vi "ReversedEngineering UpdateClassMethods.vi"(1 "ClassPath/LvClassRef":variant, 2 "Methods":string[](array[string]), 5 "error in (no error)":errorcluster, 6 "BaseClass":bool, 7 "Don'tShowDialog(False)":bool, 8 "UseVirtualMethods(True)":bool=TRUE) -> (19 "error out":errorcluster)   [LabVIEW 2012]
uses:
  <resource>/Framework/Providers/Open_GDS/ClassProviders/Provider_BaseClassInterface/ClassReader_class/ClassReader.lvclass
  <resource>/Framework/Providers/Open_GDS/ClassProviders/Provider_LvNativeClass/ClassWriterNative_class/ClassWriterNative.lvclass
  <resource>/Framework/Providers/Open_GDS/ClassProviders/Provider_BaseClassInterface/CreateMethodData.ctl
  <resource>/Framework/Providers/Open_GDS/ClassProviders/Provider_EndevoGOOP300/GOOP300_SubVIs/GOOP300_MethodScopeType.ctl
  <resource>/Framework/Providers/Open_GDS/ClassProviders/Provider_LvNativeClass/ClassWriterNative_class/IconDetails.ctl
  <resource>/Framework/Providers/Open_GDS/ClassProviders/Provider_LvNativeClass/ClassWriterNative_class/IconSize.ctl
  <resource>/Framework/Providers/Open_GDS/ClassProviders/Provider_BaseClassInterface/ClassWriter_class/ClassWriter.lvclass
panel:
  out "Creating methods":u8(slide) scale=0.0..100.0
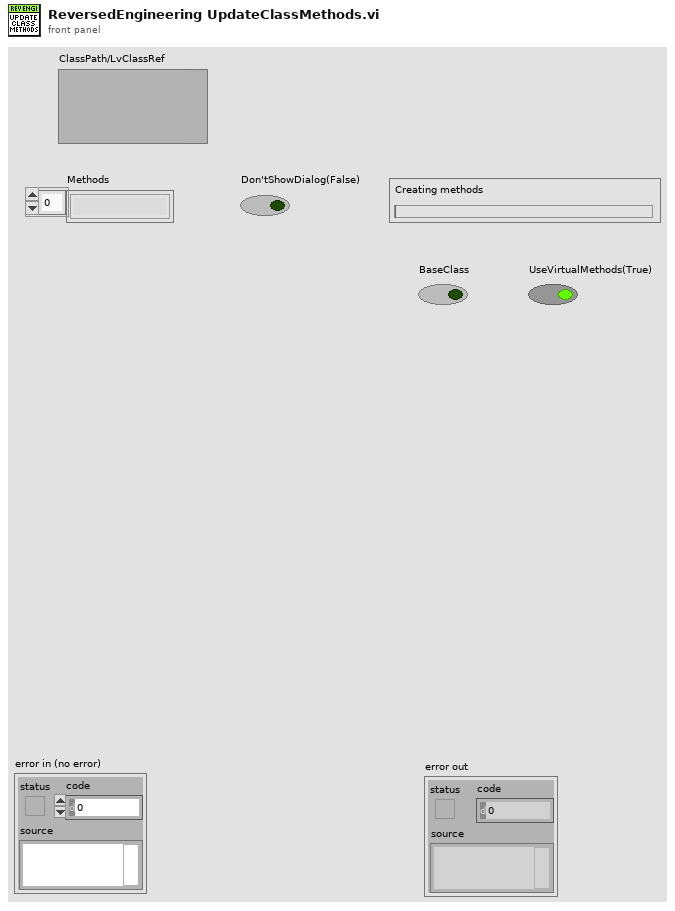
[diagram p1: front panel]
types:
  T1 = cluster{"Methods":cluster{"MethodName":string, "Private":bool, "Virtual":bool, "Reentrant":bool, "Description":string, "Icon Method Name":string, "Protected":bool, "Method Type":enum16{"Get", "Set", "GetProperty", "SetProperty"}, "Attribute":string, "ClassAtt":bool}[], "MethodPaths":path[], "MethodPrivate":bool[], "ClassItemRef":refnum<vi>}
  T2 = cluster{"MethodName":string, "Private":bool, "Virtual":bool, "Reentrant":bool, "Description":string, "Icon Method Name":string, "Protected":bool, "Method Type":enum16{"Get", "Set", "GetProperty", "SetProperty"}, "Attribute":string, "ClassAtt":bool}
  T3 = cluster{"MethodName":string, "Private":bool, "Virtual":bool, "Reentrant":bool, "Description":string, "Icon Method Name":string, "Protected":bool, "Method Type":enum16{"Get", "Set", "GetProperty", "SetProperty"}, "Attribute":string, "ClassAtt":bool}[]
  T4 = enum16{"Get", "Set", "GetProperty", "SetProperty"}
  T5 = typedef "ClassWriter.lvclass/CreateMethodData.ctl" = cluster{"MethodName":string, "RelativeMethodPath":path, "MethodDescription":string, "Scope/Visibility":T6, "MethodTemplateName":string, "IconOut":u8[][], "RelativeProjectClassPath":string, "OpenViAfterCreation":bool, "DynamicDispatchVi":bool, "ExtraCreateParameters":variant, "MustOverride":bool, "MustCallParent":bool, "IconDetails":T7, "AF-Option":variant, "TemplatePath":path}
  T6 = typedef "GOOP300_MethodScopeType.ctl" = enum16{"Use Parent Folder Scope", "Public", "Protected", "Private", "Community"}
  T7 = typedef "ClassWriterNative.lvclass/IconDetails.ctl" = cluster{"IconSize":T8, "ImageRows(32)":i32, "ConnectorPaneHeight":i32[]}
  T8 = typedef "ClassWriterNative.lvclass/IconSize.ctl" = enum16{"Full", "1 c-term high", "2 c-term high", "3 c-term high"}
  T9 = cluster{"AttributeNames":string[], "PropertyNode":bool, "FolderNames":string[]}
  T10 = typedef "ClassTypes_MethodType.ctl" = cluster{"MethodName":string, "Visibility":enum16{"Public", "Private", "Protected"}, "StereoType":string, "Path":path}
  T11 = typedef "ReversedEngineering AttributeInfoType.ctl" = cluster{"name":string, "type":T12, "dimension":i32, "typeName":string, "typePath":path, "visibility":T13}
  T12 = typedef "CommonVIs_AttributeDataType.ctl" = enum16{"UINT8", "INT8", "UINT16", "INT16", "UINT32", "INT32", "UINT64", "INT64", "SGL", "DBL", "EXT", "CSG", "CDB", "CXT", "TimeStamp", "STRING", "PATH", "BOOL", "ENUM", "RefNum", "VIRefNum", "LabVIEW Class", "Cluster", "Variant", "TypeDef", "Waveform", "LabVIEW Object", "Other", "void"}
  T13 = typedef "UMLEditor_VisibilityType.ctl" = enum16{"Public", "Private", "Protected"}
  T14 = typedef "GDSLvCLass_ClassSettingsType.ctl" = cluster{"ClassProviderName":string, "ClassTemplateUsed":string, "ClassTemplateVersion":string, "ClassDescription":string, "PlugIns":T15[], "ConnectorPanePattern":string}
  T15 = typedef "GDSLvClass_PlugIn.ctl" = cluster{"Type":T16, "ID":string, "Version":string, "Path":path, "Name":string, "Data":variant}
  T16 = typedef "GDSLvClass_PlugInTypes.ctl" = enum16{"DesignPattern", "MethodTypes"}
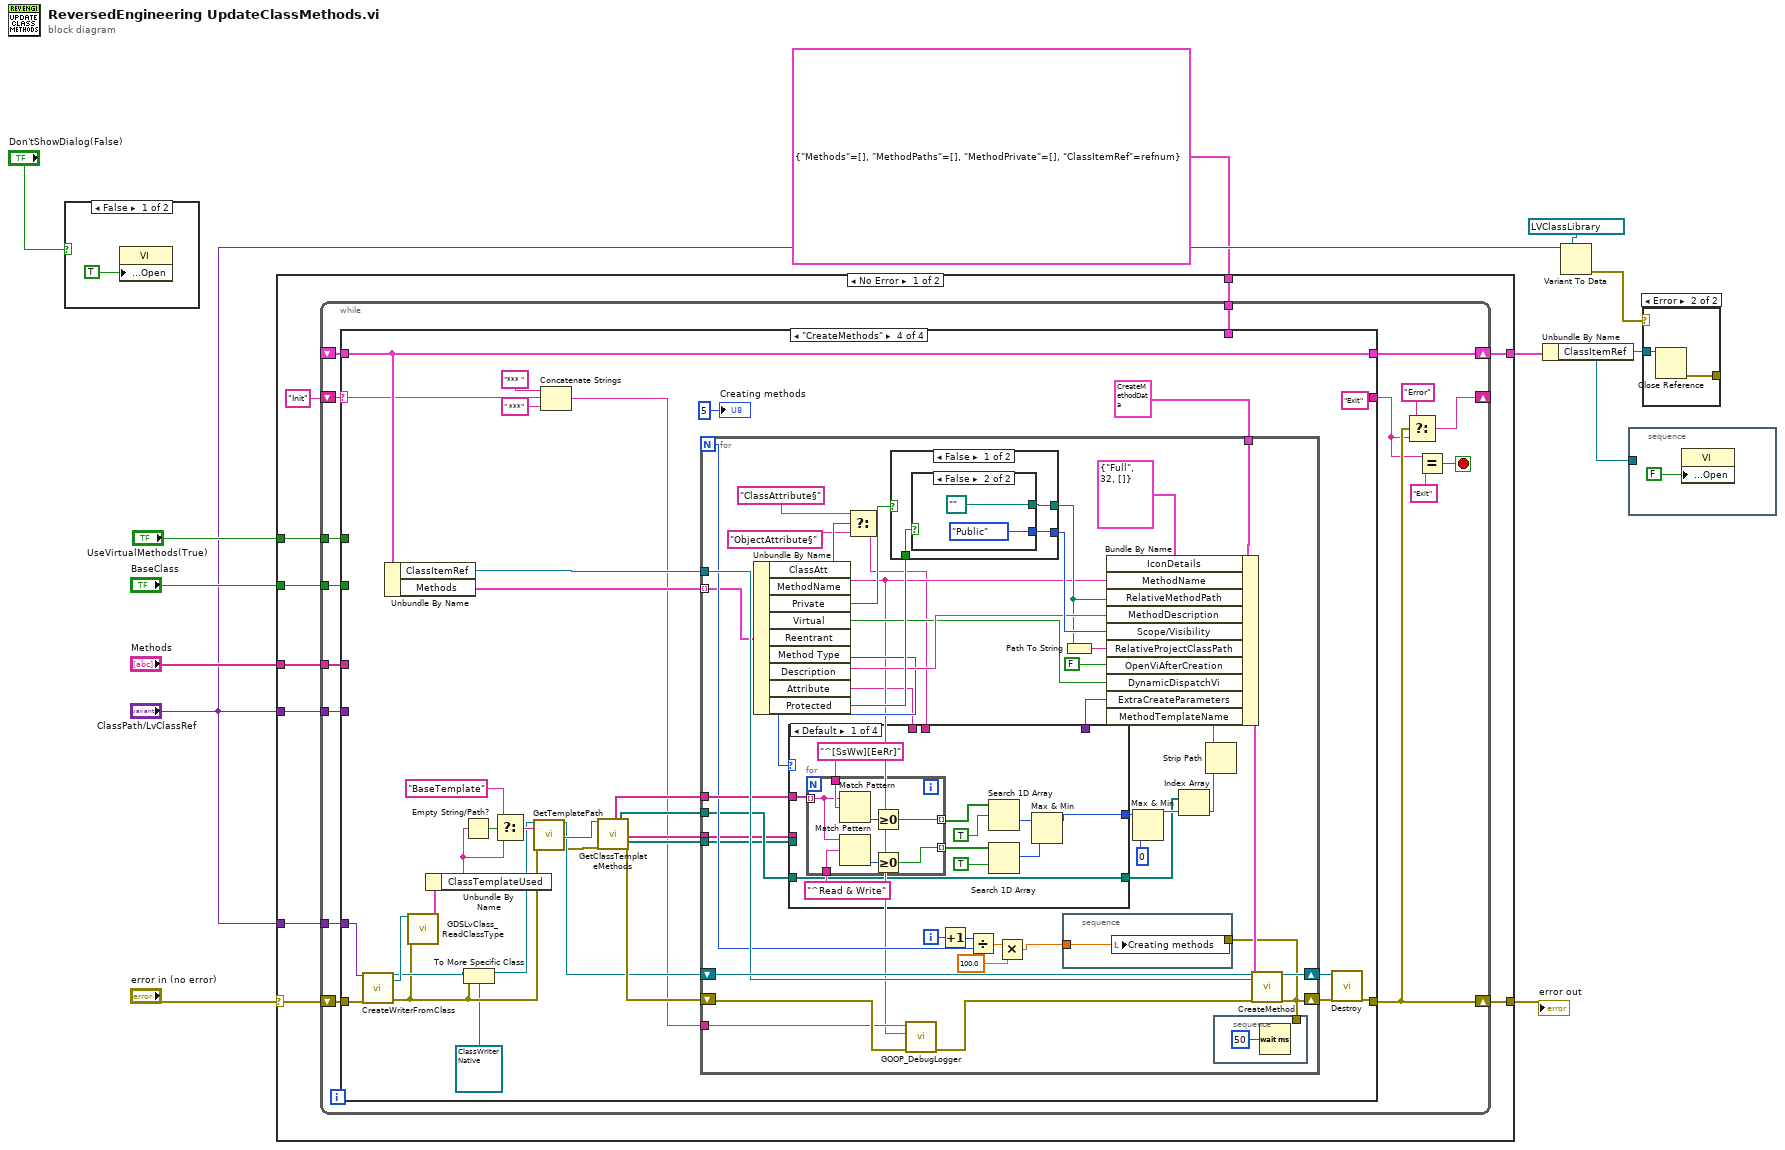
[diagram p0: block diagram]
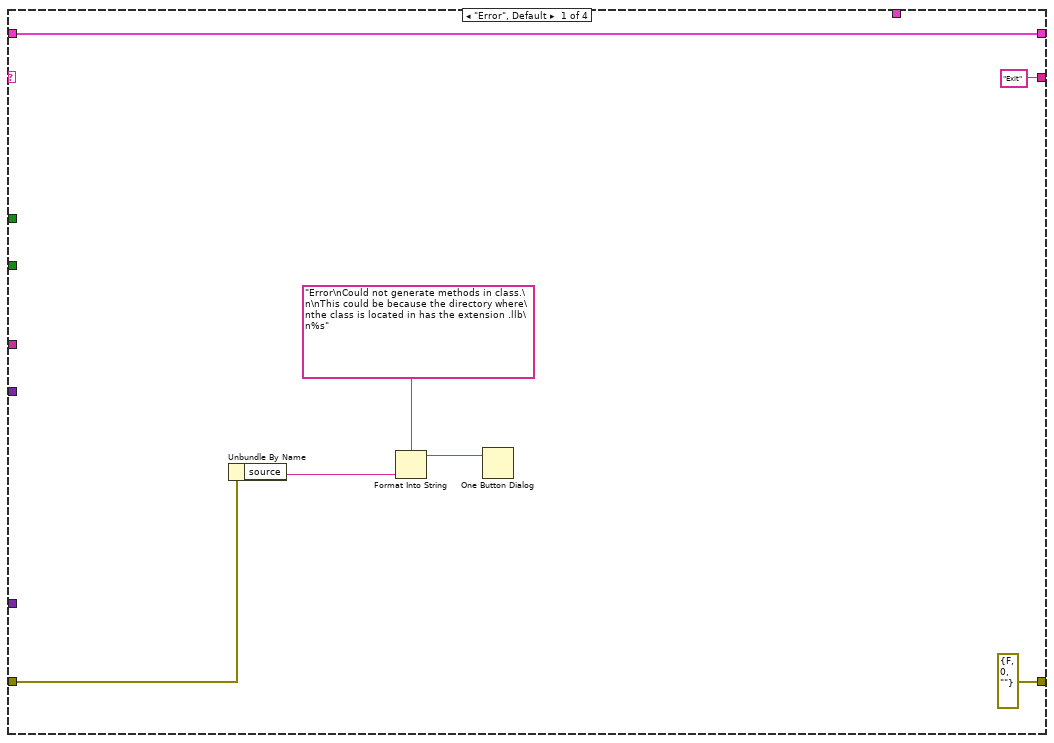
[diagram p4: hidden frame]
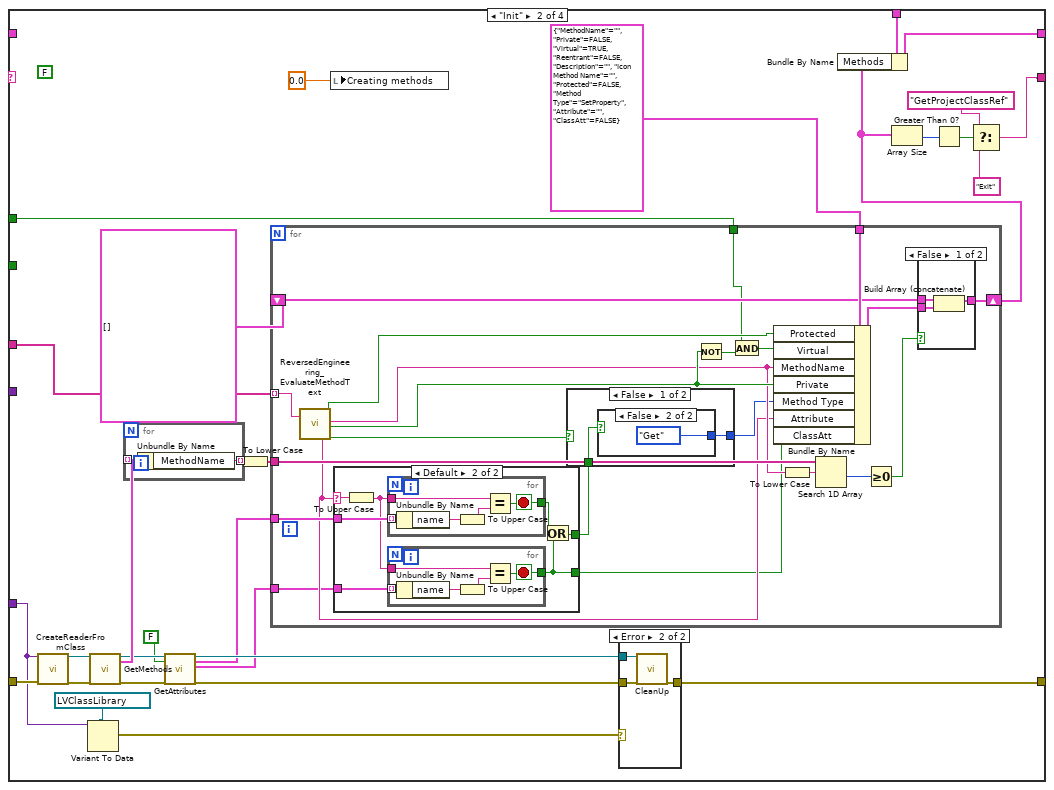
[diagram p5: hidden frame]
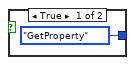
[diagram p8: hidden frame]
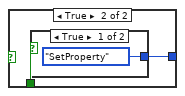
[diagram p9: hidden frame]
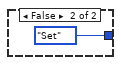
[diagram p10: hidden frame]
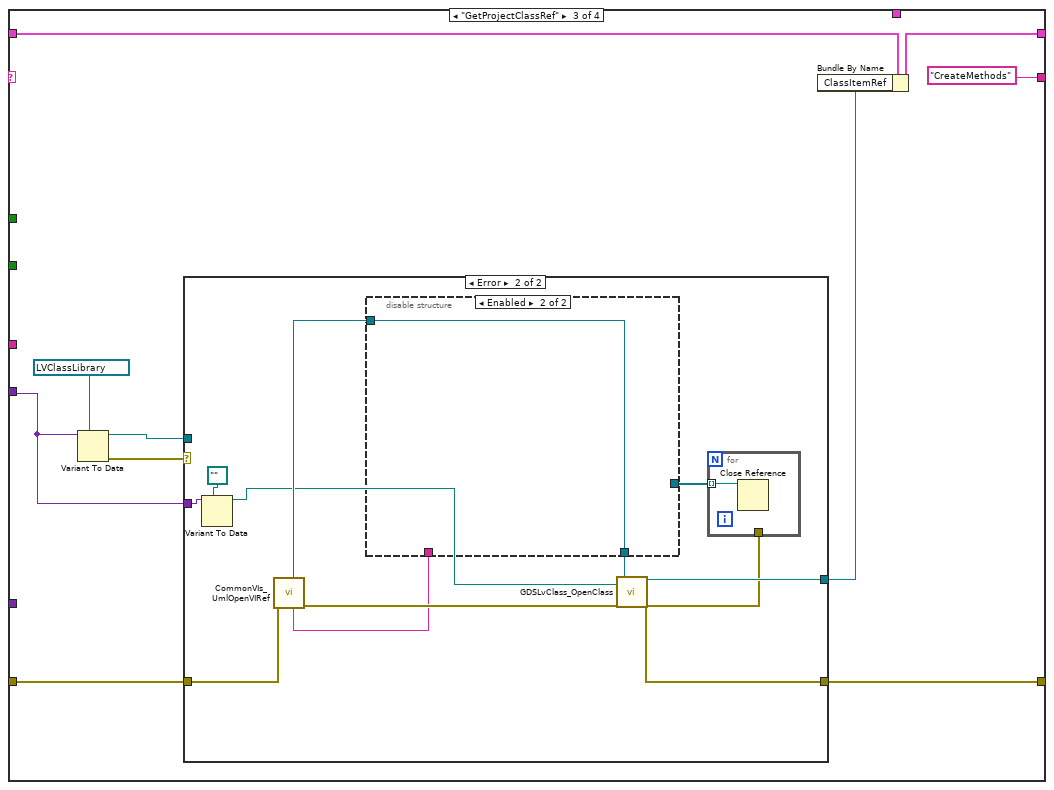
[diagram p12: hidden frame]
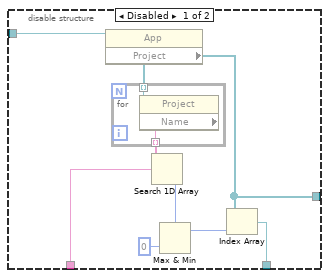
[diagram p14: hidden frame]
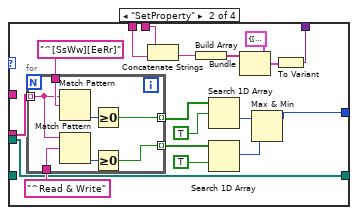
[diagram p15: hidden frame]
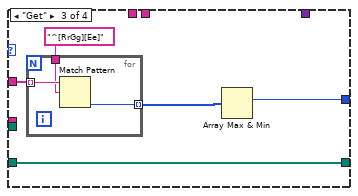
[diagram p16: hidden frame]
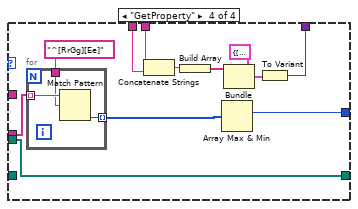
[diagram p17: hidden frame]
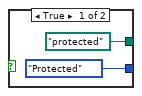
[diagram p18: hidden frame]
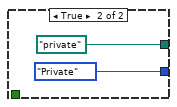
[diagram p19: hidden frame]
diagram:
  n1 = case shown="False" "Don'tShowDialog(False)" {
    frame False {
      n2 = property class="VI"("Front Panel.Open"=TRUE ("Front Panel Window:Open")) -> ()  [unwired: 2 in, 2 out]
    }
    frame True {
    }
  }
  n3 = case shown="No Error" "error in (no error)" {
    selector: "error in (no error)" -> [w23 w321]
    tunnel: [w22 w321] -> w10
    tunnel: "ClassPath/LvClassRef" -> [w20 _]
    tunnel: "Methods" -> [w19 _]
    tunnel: "ClassPath/LvClassRef" -> [w18 _]
    tunnel: [w17 _] -> w9
    tunnel: "BaseClass" -> [w16 _]
    tunnel: "UseVirtualMethods(True)" -> [w15 _]
    tunnel: T1 {"Methods"=[], "MethodPaths"=[], "MethodPrivate"=[], "ClassItemRef"=refnum} -> [w14 _]
    frame No Error {
      n4 = while {
        shift-right: [w32] -> w22
        shift-left: w23 -> [w38]
        shift-right: [w33] -> _
        shift-left: "Init" -> [w39]
        tunnel: w20 -> [w37]
        shift-right: [w36] -> w17
        shift-left: _ -> [w35]
        tunnel: w19 -> [w28]
        tunnel: w18 -> [w27]
        tunnel: w16 -> [w26]
        tunnel: w15 -> [w25]
        tunnel: w14 -> [w24]
        stop <- w29 stop-if-true
        n5 = case shown="\"CreateMethods\"" w39 {
          selector: w39 -> [_ _ _ w172]
          tunnel: w38 -> [w43 w58 w140 w198]
          tunnel: w37 -> [_ w56 _ w180]
          tunnel: ["Exit" ("y") w68 "CreateMethods" ("y") "Exit" ("y")] -> w31
          tunnel: [w45 w76 w141 w177] -> w36
          tunnel: [errorcluster {"status"=FALSE, "code"=0, "source"=""} ("error out") w65 w138 w178] -> w32
          tunnel: w35 -> [w45 _ w142 w177]
          tunnel: w28 -> [_ w75 _ _]
          tunnel: w27 -> [_ _ w136 _]
          tunnel: w26 -> [_ _ _ _]
          tunnel: w25 -> [_ w60 _ _]
          tunnel: w24 -> [_ w49 _ _]
          frame "Error", Default {
            n6 = Unbundle By Name(w43) -> ("source"=w42:string)
            n7 = Format Into String(format string="Error\nCould not generate methods in class.\n\nThis could be because the directory where\nthe class is located in has the extension .llb\n%s" ("message"), w42) -> (resulting string=w41:string)  [unwired: 2 in, 1 out]
            n8 = One Button Dialog(message=w41) -> ()  [unwired: 2 out]
          }
          frame "Init" {
            (unwired) FALSE
            n9 = call <resource>:"CreateReaderFromClass.vi"("ClassPath/LvClassRef"=w56, "error in"=w58) -> ("ClassReader"=w67:refnum<class "ClassReader.lvclass">, "error out"=w66:errorcluster)  [unwired: 16 out]
            n10 = Variant To Data(type=refnum<vi> refnum ("LVClass.Open"), Variant=w56) -> (error out=w55:errorcluster)  [unwired: 1 in, 1 out]
            n11 = call-dynamic "GetMethods.vi"("ClassReader in"=w67, "error in (no error)"=w66) -> ("ClassReader out"=w54:refnum<class "ClassReader.lvclass">, "Methods"=w64:T10[], "error out"=w53:errorcluster)  [unwired: 15 out]
            n12 = for {
              tunnel: w64 -> [w82] mode=indexing
              tunnel: [w81] -> w63 mode=indexing
              n13 = Unbundle By Name(w82) -> ("MethodName"=w81:string)
            }
            n14 = call-dynamic "GetAttributes.vi"("ClassReader in"=w54, "OnlyGetReference"=FALSE, "error in (no error)"=w53) -> ("ClassReader out"=w52:refnum<class "ClassReader.lvclass">, "ObjectAttributes"=w48:T11[], "ClassAttributes"=w47:T11[], "error out"=w51:errorcluster)  [unwired: 11 in, 2 out]
            n15 = To Lower Case(string=w63) -> (all lower case string=w62:string[])
            n16 = for {
              tunnel: w75 -> [w91] mode=indexing
              tunnel: T2 {"MethodName"="", "Private"=FALSE, "Virtual"=TRUE, "Reentrant"=FALSE, "Description"="", "Icon Method Name"="", "Protected"=FALSE, "Method Type"=enum."SetProperty", "Attribute"="", "ClassAtt"=FALSE} ("element") -> [w104]
              shift-right: [w103] -> w73
              shift-left: T3 [] -> [w102]
              tunnel: w62 -> [w99]
              tunnel: w60 -> [w92]
              tunnel: w48 -> [w87]
              tunnel: w47 -> [w84]
              n17 = call <resource>:"ReversedEngineering_EvaluateMethodText.vi"("String"=w91) -> ("MethodAttributeName"=w85:string, "Protected"=w96:bool, "MethodName"=w90:string, "Private"=w94:bool, "SetMethod"=w89:bool)  [unwired: 1 in, 13 out]
              n18 = case shown="Default" w85 {
                selector: w85 -> [_ w110]
                tunnel: w87 -> [_ w111]
                tunnel: [_ w106] -> w86
                tunnel: w84 -> [_ w108]
                tunnel: [_ w105] -> w83
                frame "" {
                }
                frame Default {
                  n19 = To Upper Case(1:w110) -> (0:w109:string)
                  n20 = for {
                    tunnel: w111 -> [w121] mode=indexing
                    tunnel: w109 -> [w118]
                    tunnel: [w117] -> w107
                    stop <- w117 stop-if-true
                    n21 = Unbundle By Name(w121) -> ("name"=w120:string)
                    n22 = To Upper Case(1:w120) -> (0:w119:string)
                    n23 = Equal?(x=w118, y=w119) -> (x = y?=w117:bool)
                  }
                  n24 = for {
                    tunnel: w108 -> [w116] mode=indexing
                    tunnel: w109 -> [w113]
                    tunnel: [w112] -> w105
                    stop <- w112 stop-if-true
                    n25 = Unbundle By Name(w116) -> ("name"=w115:string)
                    n26 = To Upper Case(1:w115) -> (0:w114:string)
                    n27 = Equal?(x=w113, y=w114) -> (x = y?=w112:bool)
                  }
                  n28 = Or(x=w107, y=w105) -> (x .or. y?=w106:bool)
                }
              }
              n29 = case shown="False" w89 {
                tunnel: [w123 w127] -> w88
                tunnel: w86 -> [w122 w126]
                frame False {
                  n30 = case shown="False" w122 {
                    tunnel: [T4."GetProperty" ("Method Type") T4."Get" ("Method Type")] -> w123
                    frame True {
                    }
                    frame False {
                    }
                  }
                }
                frame True {
                  n31 = case shown="True" w126 {
                    tunnel: [T4."SetProperty" ("Method Type") T4."Set" ("Method Type")] -> w127
                    frame True {
                    }
                    frame False {
                    }
                  }
                }
              }
              n32 = Not(x=w94) -> (.not. x?=w95:bool)
              n33 = And(x=w92, y=w95) -> (x .and. y?=w93:bool)
              n34 = Bundle By Name(cluster=w104, "Protected"=w96, "Virtual"=w93, "MethodName"=w90, "Private"=w94, "Method Type"=w88, "Attribute"=w85, "ClassAtt"=w83) -> (w101:T2)
              n35 = To Lower Case(string=w90) -> (all lower case string=w100:string)
              n36 = Search 1D Array(1D array=w99, element=w100) -> (index of element=w98:i32)  [unwired: 1 out]
              n37 = Greater Or Equal To 0?(x=w98) -> (x >= 0?=w97:bool)
              n38 = case shown="False" w97 {
                tunnel: [w132 w133] -> w103
                tunnel: w102 -> [w131 w133]
                tunnel: w101 -> [w130 _]
                frame False {
                  n39 = Build Array (concatenate)(w131, w130) -> (w132:T3)
                }
                frame True {
                }
              }
            }
            n40 = local write "Creating methods"(0.0 ("Methods (%)")) -> ()
            n41 = case shown="Error" w55 {
              tunnel: w51 -> [w77 w80]
              tunnel: w52 -> [_ w79]
              tunnel: [w77 w78] -> w65
              frame No Error {
              }
              frame Error {
                n42 = call-dynamic "CleanUp.vi"("reference in"=w79, "error in (no error)"=w80) -> ("error out"=w78:errorcluster)  [unwired: 17 out]
              }
            }
            n43 = Bundle By Name(cluster=w49, "Methods"=w73) -> (w76:T1)
            n44 = Array Size(array=w73) -> (size(s)=w72:i32)
            n45 = Greater Than 0?(x=w72) -> (x > 0?=w71:bool)
            n46 = Select(t="GetProjectClassRef" ("y"), s=w71, f="Exit" ("y")) -> (s? t:f=w68:string)
          }
          frame "GetProjectClassRef" {
            n47 = Variant To Data(type=refnum<vi> refnum ("LVClass.Open"), Variant=w136) -> (data=w134:refnum<vi>, error out=w135:errorcluster)  [unwired: 1 in]
            n48 = case shown="Error" w135 {
              tunnel: w140 -> [w144 w152]
              tunnel: [w145 w151] -> w139
              tunnel: [w144 w146] -> w138
              tunnel: w136 -> [_ w149]
              tunnel: w134 -> [w145 _]
              frame No Error {
              }
              frame Error {
                n49 = Variant To Data(type=path "", Variant=w149) -> (data=w148:path)  [unwired: 1 in, 1 out]
                n50 = call <resource>:"CommonVIs_UmlOpenVIRef.vi"("error in"=w152) -> ("error out"=w156:errorcluster, "ProjectNameOut"=w154:string, "AppRefOut"=w155:refnum<vi>)  [unwired: 3 in, 5 out]
                n51 = disable-structure shown="Enabled" {
                  disable-tunnel: w155 -> [w160 w167]
                  disable-tunnel: w154 -> [w159 _]
                  disable-tunnel: [w158 w167] -> w153
                  disable-tunnel: [w157 _] -> w147
                  frame Disabled {
                    n52 = property class="App"(reference=w160) -> ("Project"=w157:refnum<vi>[])  [unwired: 1 in, 2 out]
                    n53 = for {
                      tunnel: w157 -> [w166] mode=indexing
                      tunnel: [w165] -> w164 mode=indexing
                      n54 = property class="Project"(reference=w166) -> ("Name"=w165:string)  [unwired: 1 in, 2 out]
                    }
                    n55 = Search 1D Array(1D array=w164, element=w159) -> (index of element=w163:i32)  [unwired: 1 out]
                    n56 = Max & Min(x=w163, y=0) -> (max(x,y)=w161:i32)  [unwired: 1 out]
                    n57 = Index Array(array=w157, index=w161) -> (element=w158:refnum<vi>)
                  }
                  frame Enabled {
                  }
                }
                n58 = call <resource>:"GDSLvClass_OpenClass.vi"("ClassToOpen"=w148, "error in (no error)"=w156, "Project/ApplicationRef(If empty, currect active project will be used)"=w153) -> ("LVClass.Open"=w151:refnum<vi>, "error out"=w146:errorcluster)  [unwired: 15 out]
                n59 = for {
                  tunnel: w147 -> [w168] mode=indexing
                  tunnel: w146 -> [_]
                  n60 = Close Reference(reference=w168) -> ()  [unwired: 1 in, 1 out]
                }
              }
            }
            n61 = Bundle By Name(cluster=w142, "ClassItemRef"=w139) -> (w141:T1)
          }
          frame "CreateMethods" {
            n62 = call <resource>:"CreateWriterFromClass.vi"("ClassPath/LvClassRef"=w180, "error in"=w198) -> ("ClassWriter"=w186:refnum<class "ClassWriter.lvclass">, "LVClassRef"=w191:refnum<vi>, "error out"=w185:errorcluster)  [unwired: 15 out]
            n63 = Unbundle By Name(w177) -> ("ClassItemRef"=w197:refnum<vi>, "Methods"=w199:T3)
            n64 = call <resource>:"GDSLvClass_ReadClassType.vi"("Class Refnum In"=w191, "error in (no error)"=w185) -> ("ClassSettings"=w194:T14)  [unwired: 17 out]
            n65 = Unbundle By Name(w194) -> ("ClassTemplateUsed"=w193:string)
            n66 = Empty String/Path?(string/path=w193) -> (empty?=w196:bool)
            n67 = To More Specific Class(target class=refnum<class "ClassWriterNative.lvclass"> refnum ("reference in"), reference=w186, error in=w185) -> (specific class reference=w183:refnum<class "ClassWriterNative.lvclass">)  [unwired: 1 out]
            n68 = Select(t="BaseTemplate", s=w196, f=w193) -> (s? t:f=w192:string)
            n69 = call-dynamic "GetTemplatePath.vi"("reference in"=w183, "ClassTemplateSubDirectory"=w192, "error in (no error)"=w185) -> ("reference out"=w182:refnum<class "ClassWriterNative.lvclass">, "MethodTemplatePathOut"=w190:path, "error out"=w176:errorcluster)  [unwired: 14 out]
            n70 = Concatenate Strings("*** " ("string"), w172, " ***" ("string")) -> (w170:string)
            n71 = call <resource>:"GetClassTemplateMethods.vi"("MethodTemplatePath"=w190, "error in"=w176) -> ("NormalMethodNames"=w188:string[], "NormalMethodPaths"=w187:path[], "PropertyMethodNames"=w175:string[], "PropertyMethodPaths"=w174:path[], "error out"=w189:errorcluster)  [unwired: 1 in, 12 out]
            n72 = for {
              N -> [w226]
              tunnel: w199 -> [w204] mode=indexing
              tunnel: w197 -> [w242]
              shift-right: [w202] -> w178
              shift-left: w189 -> [w218]
              tunnel: w188 -> [w236]
              tunnel: w187 -> [w214]
              shift-right: [w221] -> w179
              shift-left: w182 -> [w243]
              tunnel: w170 -> [w216]
              tunnel: w175 -> [w212]
              tunnel: w174 -> [w211]
              tunnel: T5 {"MethodName"="", "RelativeMethodPath"=path "", "MethodDescription"="", "Scope/Visibility"=enum."Use Parent Folder Scope", "MethodTemplateName"="", "IconOut"=[], "RelativeProjectClassPath"="", "OpenViAfterCreation"=FALSE, "DynamicDispatchVi"=FALSE, "ExtraCreateParameters"=variant, "MustOverride"=FALSE, "MustCallParent"=FALSE, "IconDetails"={"IconSize"=enum."Full", "ImageRows(32)"=0, "ConnectorPaneHeight"=[]}, "AF-Option"=variant, "TemplatePath"=path ""} ("CreateMethodData") -> [w203]
              i -> [w227]
              n73 = Unbundle By Name(w204) -> ("ClassAtt"=w208:bool, "MethodName"=w215:string, "Private"=w240:bool, "Virtual"=w230:bool, "Method Type"=w219:T4, "Description"=w237:string, "Attribute"=w209:string, "Protected"=w238:bool)  [unwired: 1 out]
              n74 = Select(t="ClassAttribute§" ("string"), s=w208, f="ObjectAttribute§" ("string")) -> (s? t:f=w205:string)
              n75 = case shown="Default" w219 {
                tunnel: w236 -> [w255 _ w292 _]
                tunnel: [w246 w272 w290 w306] -> w235
                tunnel: w214 -> [w245 _ w288 _]
                tunnel: [w245 w270 w288 w303] -> w213
                tunnel: w212 -> [_ w271 _ w304]
                tunnel: w211 -> [_ w270 _ w303]
                tunnel: w209 -> [_ w269 _ w302]
                tunnel: [_ w263 _ w296] -> w210
                tunnel: w205 -> [_ w268 _ w301]
                frame Default {
                  n76 = for {
                    tunnel: w255 -> [w258] mode=indexing
                    tunnel: "^[SsWw][EeRr]" -> [w262]
                    tunnel: [w260] -> w250 mode=indexing
                    tunnel: "^Read & Write" -> [w257]
                    tunnel: [w256] -> w252 mode=indexing
                    n77 = Match Pattern(string=w258, regular expression=w262) -> (offset past match=w261:i32)  [unwired: 4 out]
                    n78 = Match Pattern(string=w258, regular expression=w257) -> (offset past match=w259:i32)  [unwired: 4 out]
                    n79 = Greater Or Equal To 0?(x=w261) -> (x >= 0?=w260:bool)
                    n80 = Greater Or Equal To 0?(x=w259) -> (x >= 0?=w256:bool)
                  }
                  n81 = Search 1D Array(1D array=w250, element=TRUE) -> (index of element=w248:i32)  [unwired: 1 out]
                  n82 = Search 1D Array(1D array=w252, element=TRUE) -> (index of element=w247:i32)  [unwired: 1 out]
                  n83 = Max & Min(x=w248, y=w247) -> (max(x,y)=w246:i32)  [unwired: 1 out]
                }
                frame "SetProperty" {
                  n84 = for {
                    tunnel: w271 -> [w283] mode=indexing
                    tunnel: "^[SsWw][EeRr]" -> [w287]
                    tunnel: [w285] -> w276 mode=indexing
                    tunnel: "^Read & Write" -> [w282]
                    tunnel: [w281] -> w278 mode=indexing
                    n85 = Match Pattern(string=w283, regular expression=w287) -> (offset past match=w286:i32)  [unwired: 4 out]
                    n86 = Match Pattern(string=w283, regular expression=w282) -> (offset past match=w284:i32)  [unwired: 4 out]
                    n87 = Greater Or Equal To 0?(x=w286) -> (x >= 0?=w285:bool)
                    n88 = Greater Or Equal To 0?(x=w284) -> (x >= 0?=w281:bool)
                  }
                  n89 = Concatenate Strings(w268, w269) -> (w264:string)
                  n90 = Build Array(w264) -> (w266:string[])
                  n91 = Search 1D Array(1D array=w276, element=TRUE) -> (index of element=w274:i32)  [unwired: 1 out]
                  n92 = Search 1D Array(1D array=w278, element=TRUE) -> (index of element=w273:i32)  [unwired: 1 out]
                  n93 = Bundle(cluster=T9 {"AttributeNames"=[], "PropertyNode"=FALSE, "FolderNames"=[]}, "AttributeNames"=w266) -> (w267:T9)  [unwired: 2 in]
                  n94 = Max & Min(x=w274, y=w273) -> (max(x,y)=w272:i32)  [unwired: 1 out]
                  n95 = To Variant(anything=w267) -> (Variant=w263:variant)
                }
                frame "Get" {
                  n96 = for {
                    tunnel: w292 -> [w295] mode=indexing
                    tunnel: "^[RrGg][Ee]" -> [w294]
                    tunnel: [w293] -> w291 mode=indexing
                    n97 = Match Pattern(string=w295, regular expression=w294) -> (offset past match=w293:i32)  [unwired: 4 out]
                  }
                  n98 = Array Max & Min(array=w291) -> (max index (indices)=w290:i32)  [unwired: 3 out]
                }
                frame "GetProperty" {
                  n99 = for {
                    tunnel: w304 -> [w310] mode=indexing
                    tunnel: "^[RrGg][Ee]" -> [w309]
                    tunnel: [w308] -> w307 mode=indexing
                    n100 = Match Pattern(string=w310, regular expression=w309) -> (offset past match=w308:i32)  [unwired: 4 out]
                  }
                  n101 = Concatenate Strings(w301, w302) -> (w297:string)
                  n102 = Build Array(w297) -> (w299:string[])
                  n103 = Array Max & Min(array=w307) -> (max index (indices)=w306:i32)  [unwired: 3 out]
                  n104 = Bundle(cluster=T9 {"AttributeNames"=[], "PropertyNode"=FALSE, "FolderNames"=[]}, "AttributeNames"=w299) -> (w300:T9)  [unwired: 2 in]
                  n105 = To Variant(anything=w300) -> (Variant=w296:variant)
                }
              }
              n106 = case shown="False" w240 {
                tunnel: [w312 path "private"] -> w228
                tunnel: [w313 GOOP300_MethodScopeType."Private" ("Scope/Visibility")] -> w239
                tunnel: w238 -> [w314 _]
                frame False {
                  n107 = case shown="False" w314 {
                    tunnel: [path "protected" path ""] -> w312
                    tunnel: [GOOP300_MethodScopeType."Protected" ("Scope/Visibility") GOOP300_MethodScopeType."Public" ("Scope/Visibility")] -> w313
                    frame True {
                    }
                    frame False {
                    }
                  }
                }
                frame True {
                }
              }
              n108 = call <resource>:"GOOP_DebugLogger.vi"("error in (no error)"=w218, "Data"=w215, "State"=w216) -> ("error out"=w217:errorcluster)  [unwired: 8 in]
              n109 = Increment(x=w227) -> (x+1=w225:i32)
              n110 = Divide(x=w225, y=w226) -> (x/y=w224:dbl)
              n111 = Multiply(x=w224, y=100.0) -> (x*y=w222:dbl)
              n112 = Path To String(path=w228) -> (string=w229:string)
              n113 = Max & Min(x=w235, y=0) -> (max(x,y)=w233:i32)  [unwired: 1 out]
              n114 = Index Array(array=w213, index=w233) -> (element=w232:path)
              n115 = Strip Path(path=w232) -> (name=w220:string)  [unwired: 1 out]
              n116 = Bundle By Name(cluster=w203, "IconDetails"=T7 {"IconSize"=enum."Full", "ImageRows(32)"=32, "ConnectorPaneHeight"=[]}, "MethodName"=w215, "RelativeMethodPath"=w228, "MethodDescription"=w237, "Scope/Visibility"=w239, "RelativeProjectClassPath"=w229, "OpenViAfterCreation"=FALSE, "DynamicDispatchVi"=w230, "ExtraCreateParameters"=w210, "MethodTemplateName"=w220) -> (w241:T5)
              n117 = call-dynamic "CreateMethod.vi"("ClassWriterNative.lvclass"=w243, "ClassItemRefIn"=w242, "CreateMethodData"=w241, "error in (no error)"=w217) -> ("ClassWriterNative.lvclass 2"=w221:refnum<class "ClassWriterNative.lvclass">, "error out"=w202:errorcluster)  [unwired: 14 out]
              n118 = stacked-sequence {
                tunnel: w202 -> [_]
                tunnel: w222 -> [w311]
                frame #0 {
                  n119 = local write "Creating methods"(w311) -> ()
                }
              }
              n120 = stacked-sequence {
                tunnel: w202 -> [_]
                frame #0 {
                  n121 = Wait (ms)(milliseconds to wait=u32 50) -> ()  [unwired: 1 out]
                }
              }
            }
            n122 = call-dynamic "Destroy.vi"("ClassWriterNative"=w179, "error in (no error)"=w178) -> ()  [unwired: 18 out]
            "Creating methods" <- u8 5 ("Creating methods")
          }
        }
        n123 = Select(t="Error", s=w32, f=w31) -> (s? t:f=w33:string)
        n124 = Equal?(x=w31, y="Exit") -> (x = y?=w29:bool)
      }
    }
    frame Error {
    }
  }
  "error out" <- w10
  n125 = Unbundle By Name(w9) -> ("ClassItemRef"=w2:refnum<vi>)
  n126 = Variant To Data(type=refnum<vi> refnum ("LVClass.Open"), Variant="ClassPath/LvClassRef") -> (error out=w4:errorcluster)  [unwired: 1 in, 1 out]
  n127 = stacked-sequence {
    tunnel: w2 -> [_]
    frame #0 {
      n128 = property class="VI"("Front Panel.Open"=FALSE ("Front Panel Window:Open")) -> ()  [unwired: 2 in, 2 out]
    }
  }
  n129 = case shown="Error" w4 {
    tunnel: w2 -> [_ w324]
    tunnel: [_ w323] -> _
    frame No Error {
    }
    frame Error {
      n130 = Close Reference(reference=w324) -> (error out=w323:errorcluster)  [unwired: 1 in]
    }
  }
